vi "BarPlot-properties.vi"(4 "MeasurementInitializationData.Measurement Names":string[](array[string]), 6 "Plot Cluster Index out":cluster{"Plot Cluster":T1, i32}, 7 "Bar graph":refnum<vi>, 8 "error in (no error)":errorcluster, 9 "color":u32[](array[colorbox]), 10 "Zen Analytics in":refnum<class "Zen Analytics.lvclass">, 11 "BarValues":dbl[][](array[numeric])) -> (0 "error out":errorcluster)   [LabVIEW 2019, in "Zen Analytics.lvlib" / "Zen Analytics.lvclass"]
uses:
  Zen Analytics.lvclass
  Dependency/GraphReff.ctl
  <vilib>/ActorFramework/Message Enqueuer/Message Enqueuer.lvclass
  Dependency/AnalyticsDataToSM.ctl
  Dependency/Plot Cluster.ctl
types:
  T1 = typedef "Zen Analytics.lvlib/Zen Analytics.lvclass/Plot Cluster.ctl" = cluster{"Reduced 2D":dbl[][], "Start Index":i32, "No Of New Termnals":i32, "Top/Bottom":bool, "Values Inserted":i32, "Re-Initialised":bool, "Statistical params":string[][], "MeasurementInitializationData":cluster{"Measurement-ID":i32[], "Measurement Names":string[], "NominalValues":dbl[], "LSL":dbl[], "USL":dbl[], "LCL":dbl[], "UCL":dbl[]}, "MeasurementData":cluster{"Measurement ID":i32, "Measurement Name":string, "Nominal Values":dbl, "LSL":dbl, "USL":dbl, "LCL":dbl, "UCL":dbl}[], "ResultData2D":dbl[][], "PlotParameters":cluster{"Trend":cluster{"TrendPlotID":dbl, "PlotProperties":cluster{"FontName":string, "FontSize":dbl, "FontColor":string, "IsBold":bool, "IsItalic":bool, "PlotColor":string}}[], "Histogram":cluster{"HistogramPlotID":dbl, "PlotProperties":cluster{"FontName":string, "FontSize":dbl, "FontColor":string, "IsBold":bool, "IsItalic":bool, "PlotColor":string}}[], "BarPlot":cluster{"BarPlotID":dbl, "BarValuesID":dbl, "PlotProperties":cluster{"FontName":string, "FontSize":dbl, "IsBold":bool, "IsItalic":bool, "FontColor":string}, "Sectors":string[]}[], "PieChart":cluster{"PieChartID":dbl, "PieChartValueID":dbl, "PlotProperties":cluster{"FontName":string, "FontSize":dbl, "IsBold":bool, "IsItalic":bool, "FontColor":string}, "Sectors":string[]}[]}}
  T2 = cluster{"BarPlotID":dbl, "BarValuesID":dbl, "PlotProperties":cluster{"FontName":string, "FontSize":dbl, "IsBold":bool, "IsItalic":bool, "FontColor":string}, "Sectors":string[]}[]
  T3 = cluster{"BarPlotID":dbl, "BarValuesID":dbl, "PlotProperties":cluster{"FontName":string, "FontSize":dbl, "IsBold":bool, "IsItalic":bool, "FontColor":string}, "Sectors":string[]}
  T4 = typedef "Zen Analytics.lvlib/Zen Analytics.lvclass/AnalyticsDataToSM.ctl" = cluster{"Actor Info":cluster{"Analytics Enqueuer":refnum<class "Message Enqueuer.lvclass">, "This VI":refnum<vi>, "Module name":string}, "Statistical Info":string[][], "Graph Refference's":T5, "ErrorMessage":string}
  T5 = typedef "Zen Analytics.lvlib/Zen Analytics.lvclass/GraphReff.ctl" = cluster{"HistgramGraph-reff":refnum<vi>[], "BarGraph-reff":refnum<vi>[], "PieGraph-reff":refnum<vi>[], "Lable-reff":refnum<vi>[], "TrendGraph-reff":refnum<vi>[], "CpCpkTable":refnum<vi>}
  T6 = cluster{"FontName":string, "FontSize":dbl, "IsBold":bool, "IsItalic":bool, "FontColor":string}
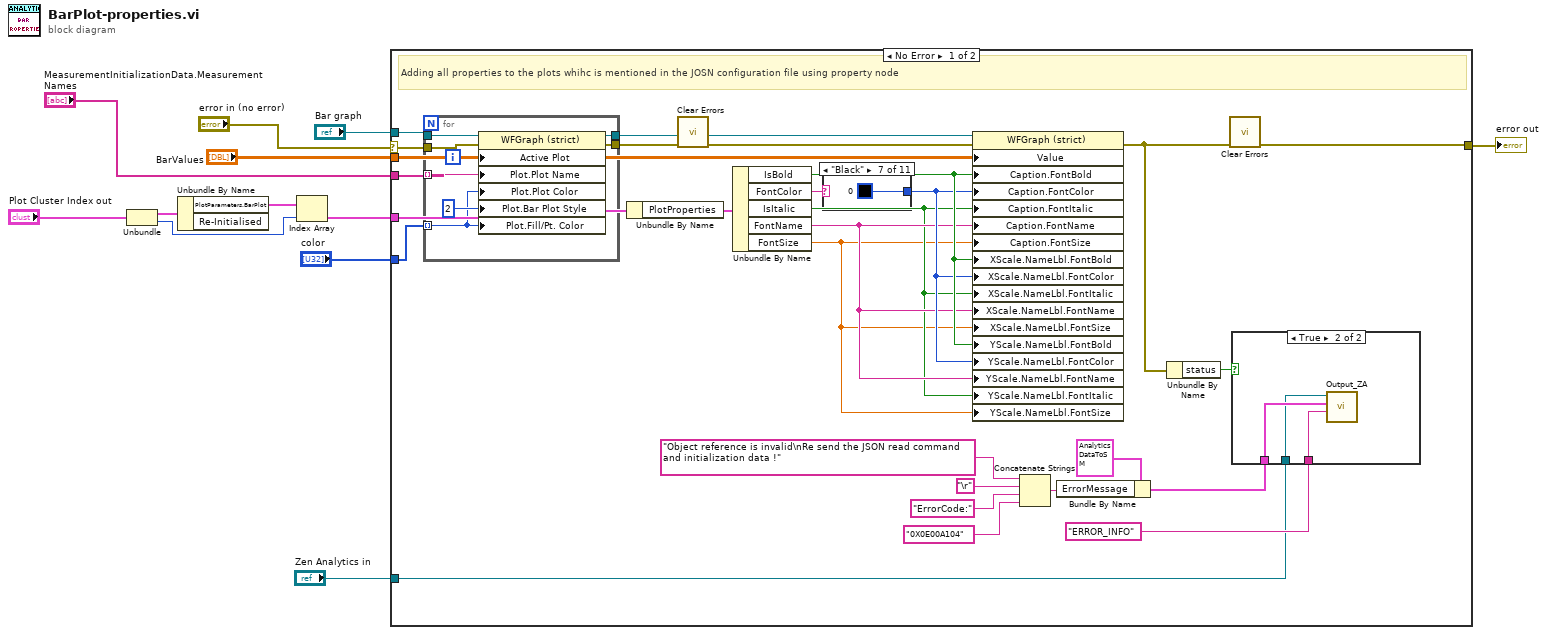
[diagram p0: block diagram]
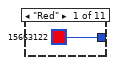
[diagram p3: hidden frame]
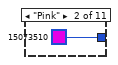
[diagram p4: hidden frame]
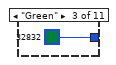
[diagram p5: hidden frame]
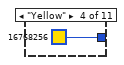
[diagram p6: hidden frame]
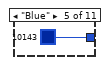
[diagram p7: hidden frame]
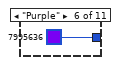
[diagram p8: hidden frame]
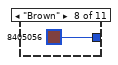
[diagram p9: hidden frame]
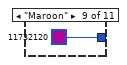
[diagram p10: hidden frame]
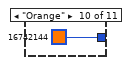
[diagram p11: hidden frame]
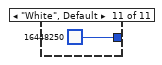
[diagram p12: hidden frame]
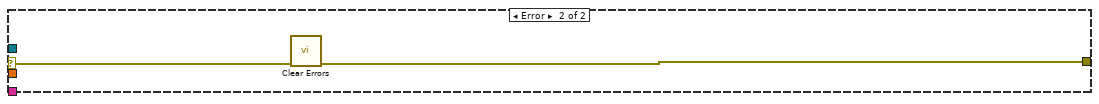
[diagram p13: hidden frame]
diagram:
  n1 = Unbundle("Plot Cluster Index out") -> ("Plot Cluster"=w10:T1, w11:i32)
  n2 = Unbundle By Name(w10) -> ("PlotParameters.BarPlot"=w9:T2)  [unwired: 1 out]
  n3 = Index Array(array=w9, index=w11) -> (element=w8:T3)
  n4 = case shown="No Error" "error in (no error)" {
    selector: "error in (no error)" -> [w38 w64]
    tunnel: w8 -> [w40 _]
    tunnel: "BarValues" -> [w39 _]
    tunnel: "Bar graph" -> [w37 _]
    tunnel: [w14 w63] -> w3
    tunnel: "color" -> [w36 _]
    tunnel: "MeasurementInitializationData.Measurement Names" -> [w35 _]
    tunnel: "Zen Analytics in" -> [w17 _]
    frame No Error {
      # "Adding all properties to the plots whihc is mentioned in the JOSN configuration file using property node"
      n5 = for {
        tunnel: [w61] -> w26
        tunnel: w38 -> [w60]
        tunnel: w35 -> [w55] mode=indexing
        tunnel: [w59] -> w27
        tunnel: w37 -> [w58]
        tunnel: w36 -> [w56] mode=indexing
        i -> [w62]
        n6 = property on="Property Node" class="WFGraph (strict)"(reference=w58, error in=w60, "Active Plot"=w62, "Plot.Plot Name"=w55, "Plot.Plot Color"=w56, "Plot.Bar Plot Style"=u8 2 ("Plot.Point Style"), "Plot.Fill/Pt. Color"=w56) -> (reference out=w59:refnum<vi>, error out=w61:errorcluster)
      }
      n7 = Unbundle By Name(w40) -> ("PlotProperties"=w33:T6)
      n8 = call <vilib>:"Clear Errors.vi"("error in (no error)"=w26) -> ("error out"=w13:errorcluster)  [unwired: 5 in, 1 out]
      n9 = Unbundle By Name(w33) -> ("IsBold"=w32:bool, "FontColor"=w34:string, "IsItalic"=w29:bool, "FontName"=w30:string, "FontSize"=w28:dbl)
      n10 = case shown="\"Black\"" w34 {
        tunnel: [u32 15663122 u32 15073510 u32 32832 u32 16768256 u32 10143 u32 7995636 u32 0 u32 8405056 u32 11732120 u32 16742144 u32 16448250] -> w31
        frame "Red" {
        }
        frame "Pink" {
        }
        frame "Green" {
        }
        frame "Yellow" {
        }
        frame "Blue" {
        }
        frame "Purple" {
        }
        frame "Black" {
        }
        frame "Brown" {
        }
        frame "Maroon" {
        }
        frame "Orange" {
        }
        frame "White", Default {
        }
      }
      n11 = property on="Property Node" class="WFGraph (strict)"(reference=w27, error in=w13, "Value"=w39, "Caption.FontBold"=w32, "Caption.FontColor"=w31, "Caption.FontItalic"=w29, "Caption.FontName"=w30, "Caption.FontSize"=w28, "XScale.NameLbl.FontBold"=w32, "XScale.NameLbl.FontColor"=w31, "XScale.NameLbl.FontItalic"=w29, "XScale.NameLbl.FontName"=w30, "XScale.NameLbl.FontSize"=w28, "YScale.NameLbl.FontBold"=w32, "YScale.NameLbl.FontColor"=w31, "YScale.NameLbl.FontName"=w30, "YScale.NameLbl.FontItalic"=w29, "YScale.NameLbl.FontSize"=w28) -> (error out=w15:errorcluster)  [unwired: 1 out]
      n12 = Concatenate Strings("Object reference is invalid\nRe send the JSON read command and initialization data !" ("SolutionForError"), "\r", "ErrorCode:", "0X0E00A104" ("ErrorCode")) -> (w20:string)
      n13 = Bundle By Name(cluster=T4 {"Actor Info"={"Analytics Enqueuer"=refnum, "This VI"=refnum, "Module name"=""}, "Statistical Info"=[], "Graph Refference's"={"HistgramGraph-reff"=[], "BarGraph-reff"=[], "PieGraph-reff"=[], "Lable-reff"=[], "TrendGraph-reff"=[], "CpCpkTable"=refnum}, "ErrorMessage"=""} ("Analytics Information"), "ErrorMessage"=w20) -> (w19:T4)
      n14 = Unbundle By Name(w15) -> ("status"=w16:bool)
      n15 = call <vilib>:"Clear Errors.vi"("error in (no error)"=w15) -> ("error out"=w14:errorcluster)  [unwired: 5 in, 1 out]
      n16 = case shown="True" w16 {
        tunnel: w19 -> [_ w43]
        tunnel: "ERROR_INFO" ("State") -> [_ w42]
        tunnel: w17 -> [_ w41]
        frame False {
        }
        frame True {
          n17 = call "Output_ZA.vi"("State"=w42, "Analytics Information"=w43, "Zen Analytics in"=w41) -> ()  [unwired: 7 in, 2 out]
        }
      }
    }
    frame Error {
      n18 = call <vilib>:"Clear Errors.vi"("error in (no error)"=w64) -> ("error out"=w63:errorcluster)  [unwired: 5 in, 1 out]
    }
  }
  "error out" <- w3
